vi "set_middle_line_states.vi"(8 "error in (no error)":errorcluster, 9 "draw y line?":bool, 10 "draw x line?":bool, 11 "Image in":refnum<class "Image.lvclass">) -> (0 "error out":errorcluster, 3 "Image out":refnum<class "Image.lvclass">)   [LabVIEW 2010, in "Image.lvclass"]
uses:
  Image.lvclass
  Image.lvclass/Image.ctl
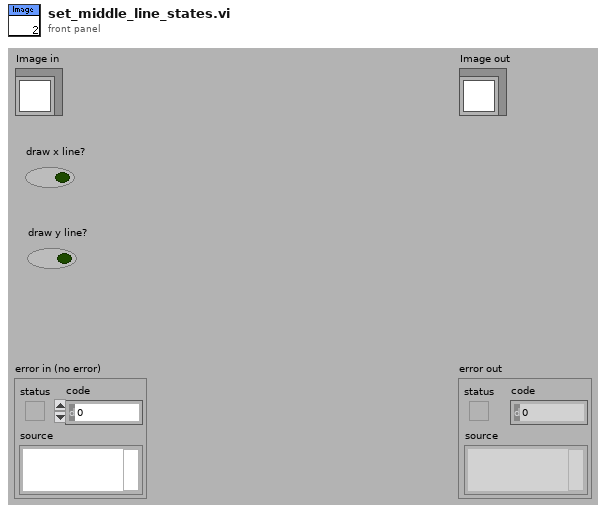
[diagram p1: front panel]
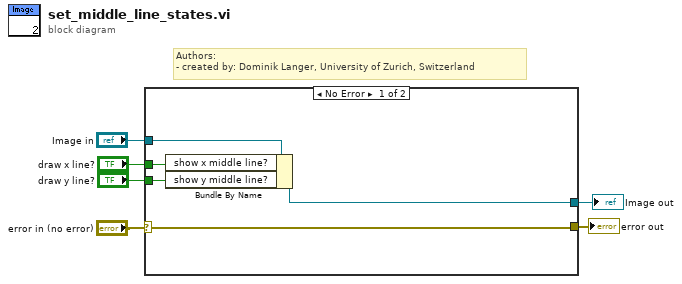
[diagram p0: block diagram]
diagram:
  # "Authors: \n- created by: Dominik Langer, University of Zurich, Switzerland"
  n1 = case shown="No Error" "error in (no error)" {
    selector: "error in (no error)" -> [w8 w13]
    tunnel: [w8 w13] -> w5
    tunnel: [w7 w12] -> w3
    tunnel: "Image in" -> [w11 w12]
    tunnel: "draw x line?" -> [w10 _]
    tunnel: "draw y line?" -> [w9 _]
    frame No Error {
      n2 = Bundle By Name(cluster=w11, "show x middle line?"=w10, "show y middle line?"=w9) -> (w7:refnum<class "Image.lvclass">)
    }
    frame Error {
    }
  }
  "error out" <- w5
  "Image out" <- w3
